vi "Table_CellValue_Tests.vi"() -> ()   [LabVIEW 2016, in "DronaTest.lvlib"]
uses:
  DronaTest.lvlib
  APIs/Stimulus/ControlValue/SetValueAuto.vi
  APIs/Stimulus/ControlValue/Controls/Listbox/SetValueByItemIndex.vi
  APIs/Assert/AssertControlValue/Equal.vi
  APIs/Stimulus/ControlValue/Controls/Table/EditCellValue.vi
  APIs/Assert/AssertControlValue/Controls/Table/AssertCellValue.vi
  <vilib>/addons/_JKI Toolkits/Caraya/classes/Assert/Assert Error.vi
  <vilib>/addons/_JKI Toolkits/Caraya/classes/Test/Test.lvclass
  <vilib>/SLL Toolkit/SLL Debug/SLL Debug.lvlib
  Drona.lvlib
  APIs/Stimulus/ControlValue/ControlValue.lvlib
  APIs/Stimulus/ControlValue/Controls/Listbox/StimulusListbox.lvlib
  APIs/Assert/AssertControlValue/AssertControlValue.lvlib
  <vilib>/addons/_JKI Toolkits/Caraya/classes/Assert/Assert.lvclass
  APIs/Stimulus/ControlValue/Controls/Table/StimulusTable.lvlib
  APIs/Assert/AssertControlValue/Controls/Table/AssertTable.lvlib
panel:
  out "error out":errorcluster
  in  "error in":errorcluster
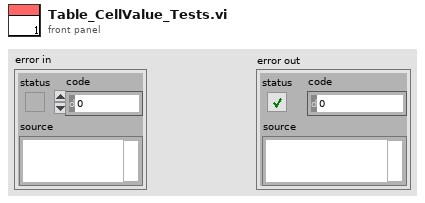
[diagram p1: front panel]
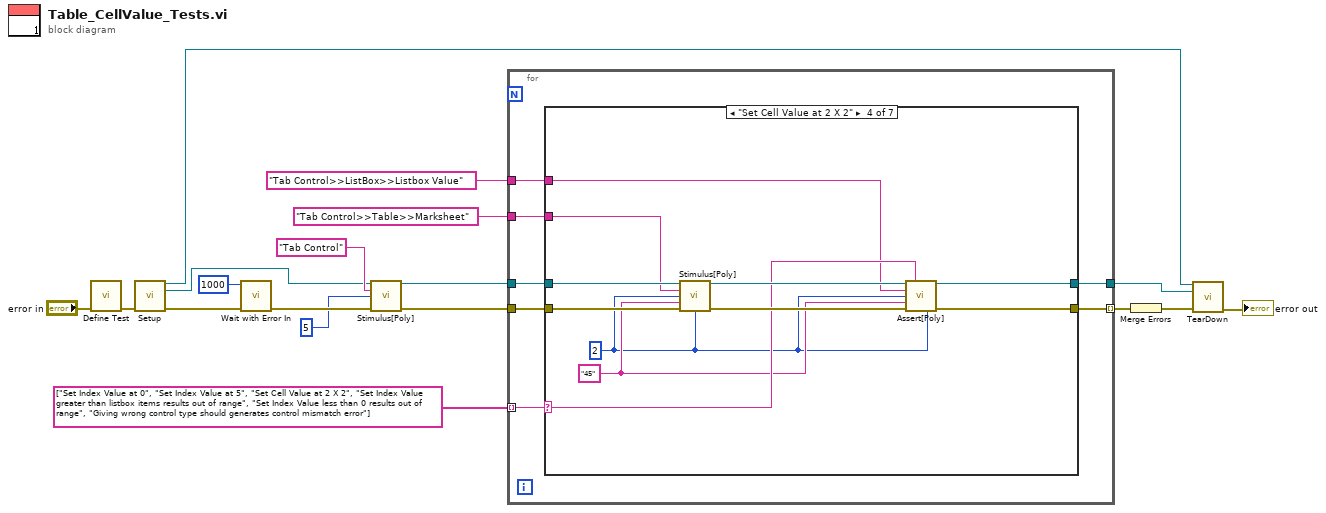
[diagram p0: block diagram]
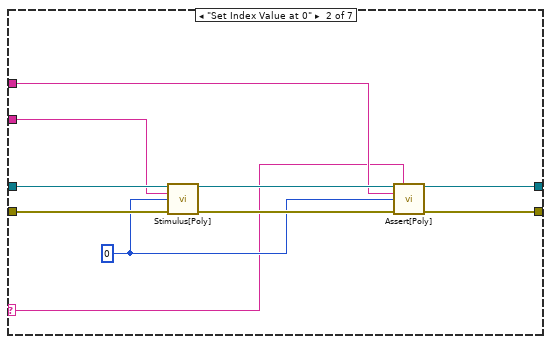
[diagram p3: hidden frame]
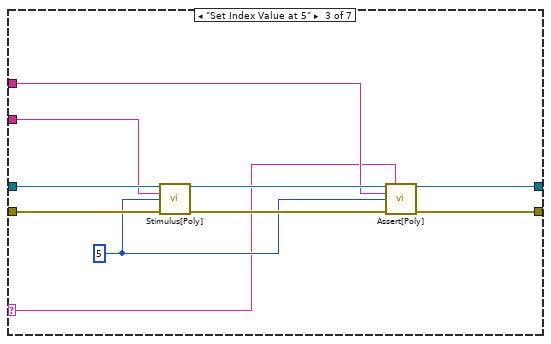
[diagram p4: hidden frame]
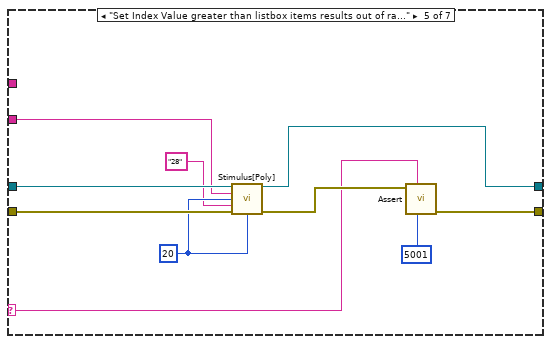
[diagram p5: hidden frame]
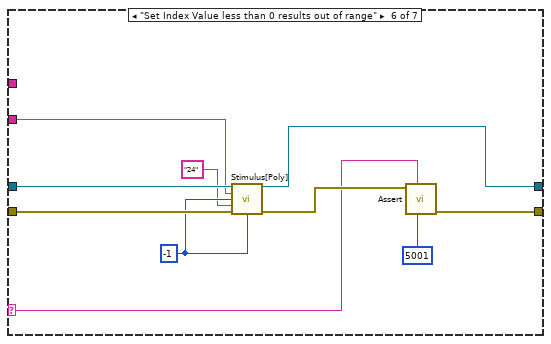
[diagram p6: hidden frame]
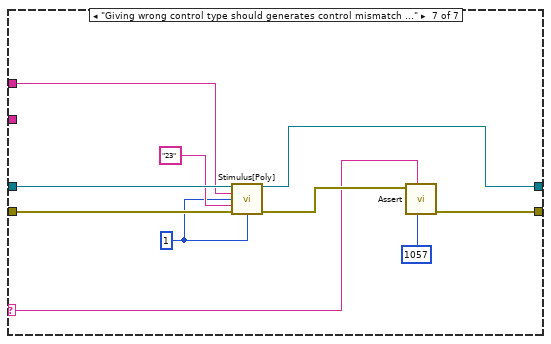
[diagram p7: hidden frame]
diagram:
  n1 = call <vilib>:"Define Test.vi"("error in (no error)"="error in") -> ("error out"=w7:errorcluster)  [unwired: 9 in, 1 out]
  n2 = call "Setup.vi"("error in (no error)"=w7) -> ("Application Ref"=w3:refnum<vi>, "VI out"=w5:refnum<vi>, "error out"=w6:errorcluster)  [unwired: 12 in]
  n3 = call <vilib>:"Wait with Error In.vi"("error in (no error)"=w6, "milliseconds to wait"=u32 1000) -> ("error out"=w16:errorcluster)  [unwired: 9 in]
  n4 = call-poly "Stimulus[Poly].vi"("VI Reference In"=w5, "Control Path"="Tab Control", "Value (Signaling)"=5, "error in"=w16) -> ("VI Reference Out"=w12:refnum<vi>, "error out"=w15:errorcluster)  [unwired: 10 in]
  n5 = for {
    tunnel: w12 -> [w24]
    tunnel: "Tab Control>>Table>>Marksheet" ("Control Path") -> [w23]
    tunnel: "Tab Control>>ListBox>>Listbox Value" ("Control Path") -> [w22]
    tunnel: string[] ["Set Index Value at 0", "Set Index Value at 5", "Set Cell Value at 2 X 2", "Set Index Value greater than listbox items results out of range", "Set Index Value less than 0 results out of range", "Giving wrong control type should generates control mismatch error"] -> [w20] mode=indexing
    tunnel: [w19] -> w2
    tunnel: w15 -> [w25]
    tunnel: [w21] -> w8 mode=indexing
    n6 = case shown="\"Set Cell Value at 2 X 2\"" w20 {
      selector: w20 -> [_ w28 w38 w52 w63 w73 w84]
      tunnel: w25 -> [w27 w37 w47 w58 w68 w78 w88]
      tunnel: w24 -> [w26 w36 w46 w57 w67 w77 w87]
      tunnel: w23 -> [_ w32 w42 w50 w66 w76 _]
      tunnel: w22 -> [_ w31 w41 w51 _ _ w81]
      tunnel: [w27 w30 w40 w54 w64 w74 w85] -> w21
      tunnel: [w26 w29 w39 w53 w61 w71 w82] -> w19
      frame Default {
      }
      frame "Set Index Value at 0" {
        w33 = 0 ("Item Index")
        n7 = call-poly "Stimulus[Poly].vi"("VI Reference In"=w36, "Control Path"=w32, "Item Index"=w33, "Error In"=w37) -> ("VI Reference Out"=w34:refnum<vi>, "Error Out"=w35:errorcluster)  [unwired: 10 in]
        n8 = call-poly "Assert[Poly].vi"("VI Reference In"=w34, "Test Label"=w28, "Control Path"=w31, "Control Value"=w33, "Error In"=w35) -> ("VI Reference Out"=w29:refnum<vi>, "Error Out"=w30:errorcluster)  [unwired: 8 in, 1 out]
      }
      frame "Set Index Value at 5" {
        w43 = 5 ("Item Index")
        n9 = call-poly "Stimulus[Poly].vi"("VI Reference In"=w46, "Control Path"=w42, "Item Index"=w43, "Error In"=w47) -> ("VI Reference Out"=w44:refnum<vi>, "Error Out"=w45:errorcluster)  [unwired: 10 in]
        n10 = call-poly "Assert[Poly].vi"("VI Reference In"=w44, "Test Label"=w38, "Control Path"=w41, "Control Value"=w43, "Error In"=w45) -> ("VI Reference Out"=w39:refnum<vi>, "Error Out"=w40:errorcluster)  [unwired: 8 in, 1 out]
      }
      frame "Set Cell Value at 2 X 2" {
        w49 = "45" ("Value")
        w48 = 2 ("Item Index")
        n11 = call-poly "Stimulus[Poly].vi"("VI Reference In"=w57, "Control Path"=w50, "Row Index"=w48, "Value"=w49, "Error In"=w58, "Column Index"=w48) -> ("VI Reference Out"=w55:refnum<vi>, "Error Out"=w56:errorcluster)  [unwired: 8 in]
        n12 = call-poly "Assert[Poly].vi"("VI Reference In"=w55, "Test Label"=w52, "Control Path"=w51, "Row Index"=w48, "Item Value"=w49, "Error In"=w56, "Column Index"=w48) -> ("VI Reference Out"=w53:refnum<vi>, "Error Out"=w54:errorcluster)  [unwired: 6 in, 1 out]
      }
      frame "Set Index Value greater than listbox items results out of range" {
        w60 = 20 ("Item Index")
        n13 = call-poly "Stimulus[Poly].vi"("VI Reference In"=w67, "Control Path"=w66, "Row Index"=w60, "Value"="28", "Error In"=w68, "Column Index"=w60) -> ("VI Reference Out"=w61:refnum<vi>, "Error Out"=w65:errorcluster)  [unwired: 8 in]
        n14 = call-poly <vilib>:"Assert.vi"("error code (1)"=5001, "Label"=w63, "Error?"=w65) -> ("error out"=w64:errorcluster)  [unwired: 7 in, 1 out]
      }
      frame "Set Index Value less than 0 results out of range" {
        w70 = -1 ("Item Index")
        n15 = call-poly "Stimulus[Poly].vi"("VI Reference In"=w77, "Control Path"=w76, "Row Index"=w70, "Value"="24", "Error In"=w78, "Column Index"=w70) -> ("VI Reference Out"=w71:refnum<vi>, "Error Out"=w75:errorcluster)  [unwired: 8 in]
        n16 = call-poly <vilib>:"Assert.vi"("error code (1)"=5001, "Label"=w73, "Error?"=w75) -> ("error out"=w74:errorcluster)  [unwired: 7 in, 1 out]
      }
      frame "Giving wrong control type should generates control mismatch error" {
        w79 = 1 ("Column Index")
        n17 = call-poly "Stimulus[Poly].vi"("VI Reference In"=w87, "Control Path"=w81, "Row Index"=w79, "Value"="23", "Error In"=w88, "Column Index"=w79) -> ("VI Reference Out"=w82:refnum<vi>, "Error Out"=w86:errorcluster)  [unwired: 8 in]
        n18 = call-poly <vilib>:"Assert.vi"("error code (1)"=1057, "Label"=w84, "Error?"=w86) -> ("error out"=w85:errorcluster)  [unwired: 7 in, 1 out]
      }
    }
  }
  n19 = Merge Errors(w8) -> (w4:errorcluster)
  n20 = call "TearDown.vi"("Application Ref"=w3, "VI in"=w2, "error in (no error)"=w4) -> ("error out"=→"error out":errorcluster)  [unwired: 12 in]
